vi "get_behaviour_flag.vi"(6 "timeout (25000ms)":i32=25000, 8 "error in (no error)":errorcluster, 9 "Read From NVM?":bool, 10 "Word Index":i64, 11 "daemon reference in":refnum<k5>) -> (0 "error out":errorcluster, 2 "response":string, 3 "daemon reference out":refnum<k5>, 5 "command out":string="random")   [LabVIEW 2017]
doc: "<b>Command: </b>\"get_behaviour_flag\"\n\n<b>Description: </b> This command returns these flag values that are stored in NVM or RAM copy.\n\n<b>Parameters: </b> Word Index, Permanent\n____________________________________________\nDIPC 692 Daemon API 10.0.0.1\nSam Tee - Dyson Technology Ltd\nCopyright (c) 2024, Dyson Technology Ltd"
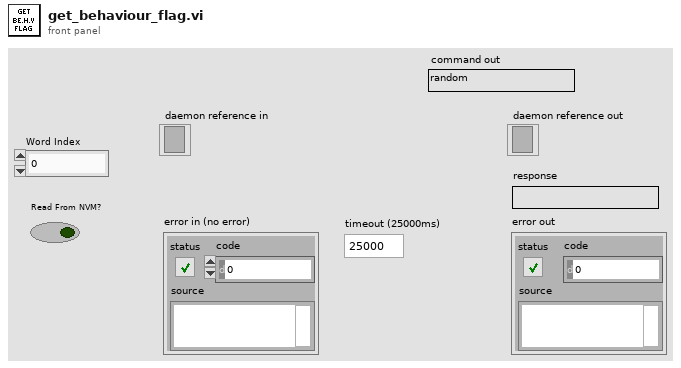
[diagram p1: front panel]
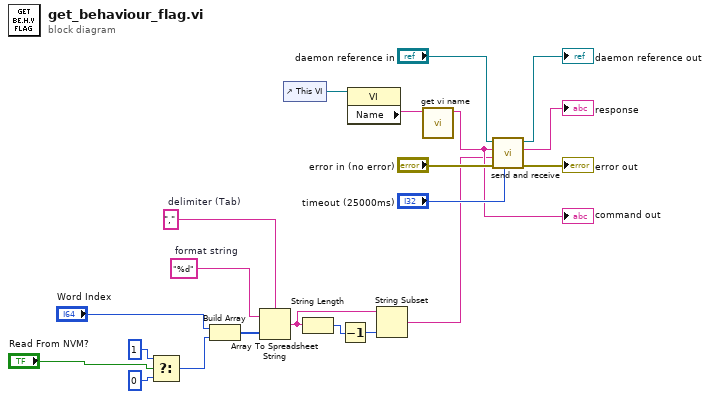
[diagram p0: block diagram]
diagram:
  w9 = ","  # delimiter (Tab)
  w12 = "%d"  # format string
  n1 = Select(t=1, s="Read From NVM?", f=0) -> (s? t:f=w1:i32)
  n2 = Build Array("Word Index", w1) -> (w6:i64[])
  n3 = Array To Spreadsheet String(delimiter (Tab)=w9, array=w6, 3:w12) -> (spreadsheet string=w5:string)
  n4 = control-ref of="This VI"() -> (w15:refnum<vi>)
  n5 = String Length(string=w5) -> (length=w11:i32)
  n6 = Decrement(x=w11) -> (x-1=w10:i32)
  n7 = property class="VI"(reference=w15) -> ("Name"=w14:string)  [unwired: 1 in, 2 out]
  n8 = String Subset(string=w5, length (rest)=w10) -> (substring=w2:string)  [unwired: 1 in]
  n9 = call "get vi name.vi"("library.lvlib:name.vi"=w14) -> ("vi name"=w13:string)  [unwired: 10 in]
  "command out" <- w13
  n10 = call "send and receive.vi"("timeout (25000ms)"="timeout (25000ms)", "error in (no error)"="error in (no error)", "data"=w2, "command"=w13, "daemon reference in"="daemon reference in") -> ("error out"=→"error out":errorcluster, "response"=→"response":string, "daemon reference out"=→"daemon reference out":refnum<k5>)  [unwired: 4 in]
